vi "Launcher.vi"   [LabVIEW 2021]
uses:
  Builder/Build object type.ctl
  GUI Builder/GUI Builder.lvclass
  Builder/Builder.lvclass
panel:
  # "Builder example"
types:
  T1 = typedef "App-Builder Library.lvlib/Builder.lvclass/Build object type.ctl" = enum16{"EXE", "RT EXE", "Deployable Packed"}
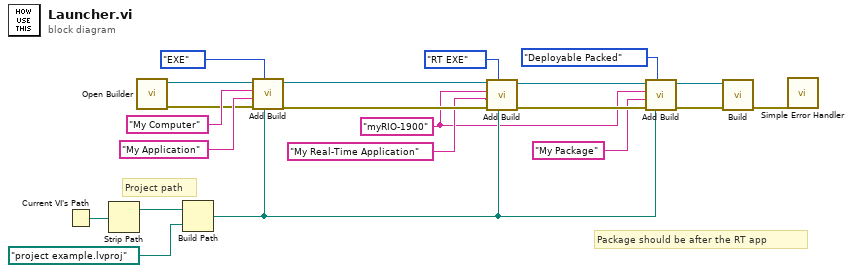
[diagram p0: block diagram]
diagram:
  w6 = "myRIO-1900" ("Target Name")
  # "Package should be after the RT app"
  # "Project path"
  n1 = Current VI's Path() -> (path=w18:path)
  n2 = Strip Path(path=w18) -> (stripped path=w17:path)  [unwired: 1 out]
  n3 = call "Open Builder.vi"() -> ("error out"=w1:errorcluster, "Builder out"=w2:refnum<class "Builder.lvclass">)  [unwired: 10 in]
  n4 = Build Path(base path=w17, name or relative path=path "project example.lvproj") -> (appended path=w8:path)
  n5 = call "Add Build.vi"("Project Path"=w8, "Build Object type"=Build_object_type."EXE", "error in (no error)"=w1, "Build Specification"="My Application" ("Target Name"), "Target Name"="My Computer", "Builder in"=w2) -> ("error out"=w20:errorcluster, "Builder out"=w21:refnum<class "Builder.lvclass">)  [unwired: 4 in]
  n6 = call "Add Build.vi"("Project Path"=w8, "Build Object type"=Build_object_type."RT EXE", "error in (no error)"=w20, "Build Specification"="My Real-Time Application" ("Target Name"), "Target Name"=w6, "Builder in"=w21) -> ("error out"=w11:errorcluster, "Builder out"=w12:refnum<class "Builder.lvclass">)  [unwired: 4 in]
  n7 = call "Add Build.vi"("Project Path"=w8, "Build Object type"=Build_object_type."Deployable Packed", "error in (no error)"=w11, "Build Specification"="My Package" ("Target Name"), "Target Name"=w6, "Builder in"=w12) -> ("error out"=w10:errorcluster, "Builder out"=w9:refnum<class "Builder.lvclass">)  [unwired: 4 in]
  n8 = call "Build.vi"("error in (no error)"=w10, "App-Builder"=w9) -> ("error out"=w19:errorcluster)  [unwired: 9 in]
  n9 = call <vilib>:"Simple Error Handler.vi"("error in (no error)"=w19) -> ()  [unwired: 4 in, 5 out]
